vi "GUI.Boolean.SetValue.vi"(7 "referenceToControls in":refnum<vi>[](array[refnum]), 8 "error in (no error)":errorcluster, 9 "booleanValue (false)":bool, 11 "booleanName":string) -> (0 "error out":errorcluster, 5 "referenceToControls out":refnum<vi>[](array[refnum]))   [LabVIEW 2019]
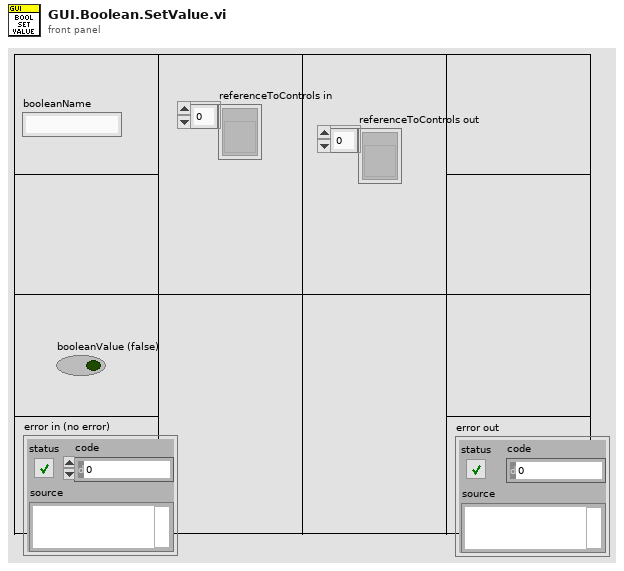
[diagram p1: front panel]
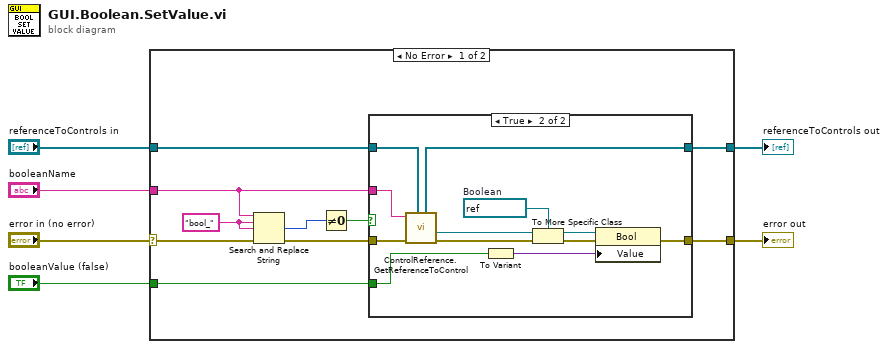
[diagram p0: block diagram]
diagram:
  n1 = case shown="No Error" "error in (no error)" {
    selector: "error in (no error)" -> [w14 w32]
    tunnel: [w16 w32] -> w5
    tunnel: "booleanName" -> [w13 _]
    tunnel: "booleanValue (false)" -> [w15 _]
    tunnel: [w8 w31] -> w3
    tunnel: "referenceToControls in" -> [w7 w31]
    frame No Error {
      w12 = "bool_"
      n2 = Search and Replace String(input string=w13, search string=w12, replace string=w12, error in=w14) -> (number of replacements=w11:i32, error out=w9:errorcluster)  [unwired: 4 in, 2 out]
      n3 = Not Equal To 0?(x=w11) -> (x != 0?=w10:bool)
      n4 = case shown="True" w10 {
        tunnel: [w18 w30] -> w16
        tunnel: w15 -> [_ w21]
        tunnel: w13 -> [_ w20]
        tunnel: w9 -> [w18 w27]
        tunnel: [w17 w25] -> w8
        tunnel: w7 -> [w17 w26]
        frame False {
        }
        frame True {
          w29 = refnum<vi> refnum  # Boolean
          n5 = call "ControlReference.GetReferenceToControl.vi"("referenceToControls in"=w26, "error in (no error)"=w27, "controlLabelText"=w20) -> ("error out"=w24:errorcluster, "referenceToControl"=w19:refnum<vi>, "referenceToControls out"=w25:refnum<vi>[])  [unwired: 6 in]
          n6 = To Variant(anything=w21) -> (Variant=w22:variant)
          n7 = To More Specific Class(target class=w29, reference=w19, error in=w24) -> (specific class reference=w28:refnum<vi>, error out=w23:errorcluster)
          n8 = property class="Bool"(reference=w28, error in=w23, "Value"=w22) -> (error out=w30:errorcluster)  [unwired: 1 out]
        }
      }
    }
    frame Error {
    }
  }
  "error out" <- w5
  "referenceToControls out" <- w3
